vi "Control.AnalysisStart.vi"(8 "Remote Path":path=path "d:/testdata/TestResults", 9 "Results Path":path=path "d:/testdata/TestResults", 10 "Temp Path":path=path "c:/testdata/temp") -> (3 "AnalysisRef":refnum<vi>)   [LabVIEW 2014, in "NIAnalysis.lvlib"]
uses:
  NIAnalysis.lvlib
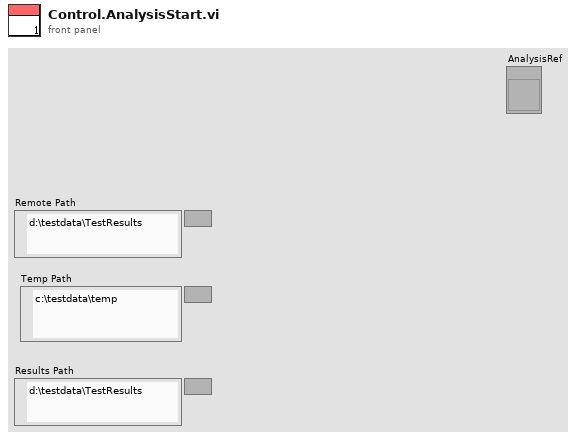
[diagram p1: front panel]
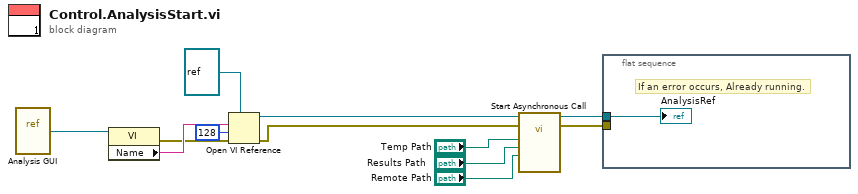
[diagram p0: block diagram]
diagram:
  n1 = vi-ref "Analysis GUI.vi"() -> (w12:refnum<vi>)
  n2 = property class="VI"(reference=w12) -> (error out=w6:errorcluster, "Name"=w11:string)  [unwired: 1 in, 1 out]
  n3 = Open VI Reference(type specifier VI Refnum (for type only)=refnum<vi> refnum, vi path=w11, options=128, error in (no error)=w6) -> (vi reference=w10:refnum<vi>, error out=w8:errorcluster)  [unwired: 2 in]
  n4 = call-by-ref "Start Asynchronous Call"(reference=w10, error in=w8, "Remote Path"="Remote Path", "Results Path"="Results Path", "Temp Path"="Temp Path") -> (reference out=w5:refnum<vi>, error out=w4:errorcluster)  [unwired: 9 in]
  n5 = flat-sequence {
    tunnel: w5 -> [w13]
    tunnel: w4 -> [_]
    frame #0 {
      # "If an error occurs, Already running."
      "AnalysisRef" <- w13
    }
  }
